vi "NewCore.vi"(8 "error in (no error)":errorcluster, 11 "Maze":refnum<class "Maze.lvclass">) -> (0 "error out":errorcluster, 3 "Maze":refnum<class "Maze.lvclass">)   [LabVIEW 2020, in "Maze.lvclass"]
uses:
  Maze.lvclass
  Private/TypeDef/privateData.ctl
  ConcreteMazeSite/Room/Room.lvclass
  Maze.lvclass/Maze.ctl
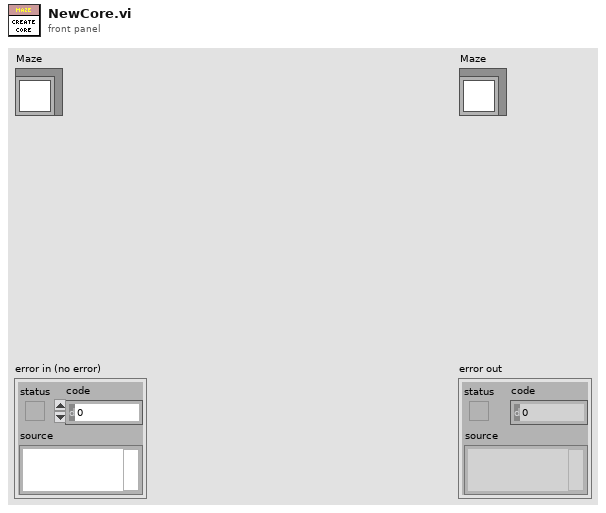
[diagram p1: front panel]
types:
  T1 = typedef "Maze.lvclass/privateData.ctl" = cluster{"mRoomVec":refnum<class "Room.lvclass">[]}
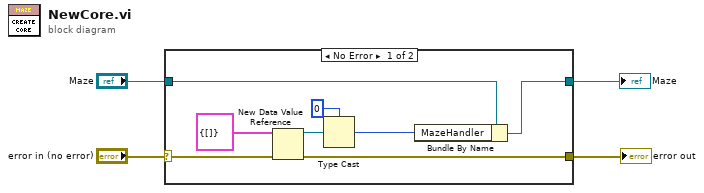
[diagram p0: block diagram]
diagram:
  n1 = case shown="No Error" "error in (no error)" {
    selector: "error in (no error)" -> [w5 w14]
    tunnel: [w8 w14] -> w4
    tunnel: [w9 w13] -> w1
    tunnel: "Maze" -> [w7 w13]
    frame No Error {
      n2 = New Data Value Reference(data value=T1 {"mRoomVec"=[]} ("privateData"), error in=w5) -> (data value reference=w12:refnum<data-value>, error out=w8:errorcluster)
      n3 = Type Cast(type=u32 0, x=w12) -> (*(type *) &x=w10:u32)
      n4 = Bundle By Name(cluster=w7, "MazeHandler"=w10) -> (w9:refnum<class "Maze.lvclass">)
    }
    frame Error {
    }
  }
  "error out" <- w4
  "Maze" <- w1
